vi "Configure Buffer Size (U32).vi"(8 "error in":errorcluster, 10 "Buffer Size":u32=1000000 format="%.0p", 11 "FPGA VI Reference":T1) -> (0 "error out":errorcluster, 3 "FPGA VI Reference":T1)   [LabVIEW 2011, in "FlexRIO Host Library (User).lvlib"]
doc: "This start acquisition by switching OFF and ON \"Arm Acquire button\".\nThis VI also starts DMA FIFO."
uses:
  FlexRIO Host Library (User).lvlib
  Session/FPGA Session Ref.ctl
  <vilib>/rvi/errors/niLvFpgaMergeErrorWithErrorCode.vi
  <vilib>/rvi/interface/nirviMethod/nirviMethod.xnode
  OCT Reference Design/FPGA Bitfiles/OCTDigitizer_FPGABoard_AcquireDatawitho_CC2D8059.lvbitx
  OCT Reference Design/Complete FPGA Engine/Acquire Data without DRAM.vi
  <vilib>/FPGAPlugInAG/PXIe-7965R/niLvFpga_ConfigureFifo_PXIe-7965R.vi
  <vilib>/FPGAPlugInAG/PXIe-7965R/niLvFpga_StartFifo_PXIe-7965R.vi
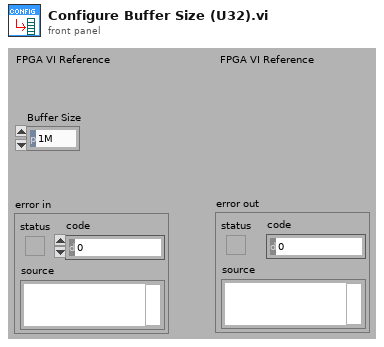
[diagram p1: front panel]
types:
  T1 = typedef "FlexRIO Host Library (User).lvlib/FPGA Session Ref.ctl" = refnum<k20>
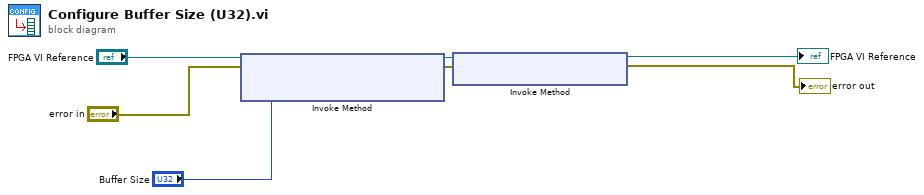
[diagram p0: block diagram]
diagram:
  n1 = xnode "Invoke Method"("FPGA VI Reference In"="FPGA VI Reference", "error in"="error in", "Depth"="Buffer Size") -> ("FPGA VI Reference Out"=w4:T1, "error out"=w3:errorcluster)
  n2 = xnode "Invoke Method"("FPGA VI Reference In"=w4, "error in"=w3) -> ("FPGA VI Reference Out"=→"FPGA VI Reference":T1, "error out"=→"error out":errorcluster)
